vi "OpenWeatherMap.vi"() -> ()   [LabVIEW 2020]
panel:
  out "main":string
  out "Humidity":dbl
  out "current time":timestamp
  out "Name":string
  out "Feels Like":dbl format="%#.1g"
  out "Temperature":dbl(slide) scale=0.0..100.0
  # "Current Weather Conditions"
  # "Igor Povarich\nRev 01/09/2021"
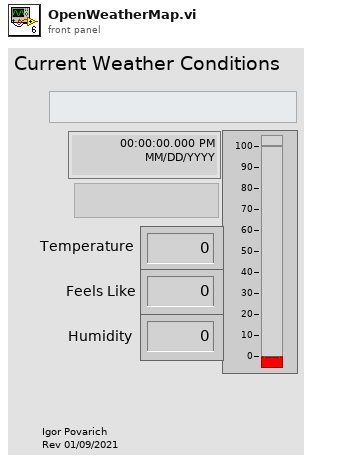
[diagram p1: front panel]
types:
  T1 = cluster{"coord":cluster{"lon":dbl, "lat":dbl}, "weather":cluster{"id":i32, "main":string, "description":string, "icon":string}[], "base":string, "main":cluster{"temp":dbl, "feels_like":dbl, "temp_min":dbl, "temp_max":dbl, "pressure":dbl, "humidity":dbl}, "visibility":i32, "wind":cluster{"speed":i32, "deg":i32}, "clouds":cluster{"all":i32}, "dt":i32, "sys":cluster{"type":i32, "id":i32, "country":string, "sunrise":i32, "sunset":i32}, "timezone":i32, "id":i32, "name":string, "cod":i32}
  T2 = cluster{"id":i32, "main":string, "description":string, "icon":string}[]
  T3 = cluster{"id":i32, "main":string, "description":string, "icon":string}
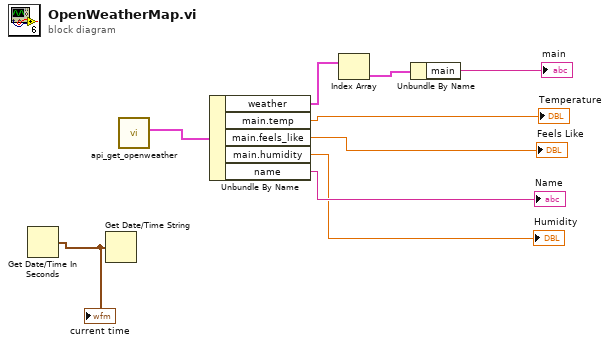
[diagram p0: block diagram]
diagram:
  n1 = Get Date/Time In Seconds() -> (seconds since 1Jan1904=w5:timestamp)
  "current time" <- w5
  n2 = Get Date/Time String(seconds (now)=w5) -> ()  [unwired: 2 in, 2 out]
  n3 = call "api_get_openweather.vi"() -> ("Cluster Out"=w9:T1)  [unwired: 9 in, 2 out]
  n4 = Unbundle By Name(w9) -> ("weather"=w3:T2, "main.temp"=→"Temperature":dbl, "main.feels_like"=→"Feels Like":dbl, "main.humidity"=→"Humidity":dbl, "name"=→"Name":string)
  n5 = Index Array(array=w3) -> (element=w2:T3)  [unwired: 1 in]
  n6 = Unbundle By Name(w2) -> ("main"=→"main":string)
